vi "Trial - Rename File.vi"(11 "Current File Name":string) -> (2 "Cancel OUT":bool, 3 "Enter New File Name OUT":string caption=".dat")   [LabVIEW 2018]
panel:
  in  "Enter New File Name":string caption=".dat"
  in  "Cancel":bool
  in  "Save":bool
  # "Enter New File Name for Trial"
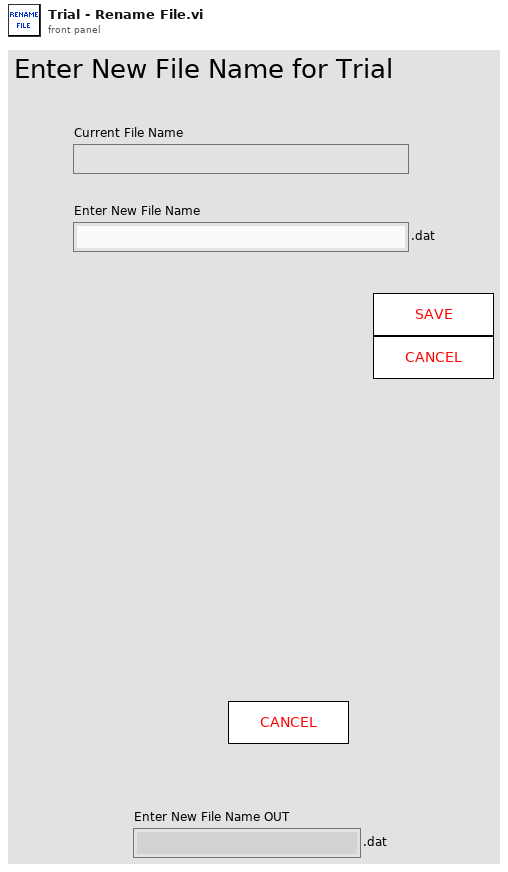
[diagram p1: front panel]
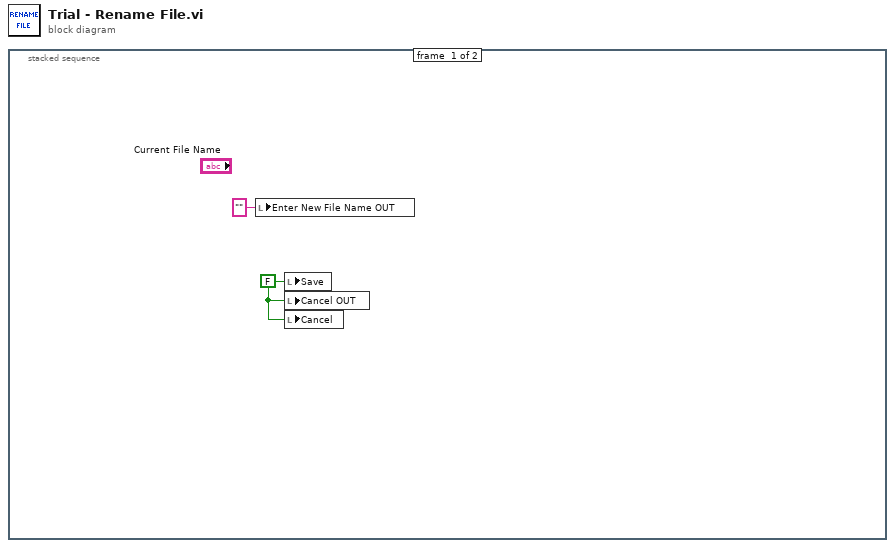
[diagram p0: block diagram]
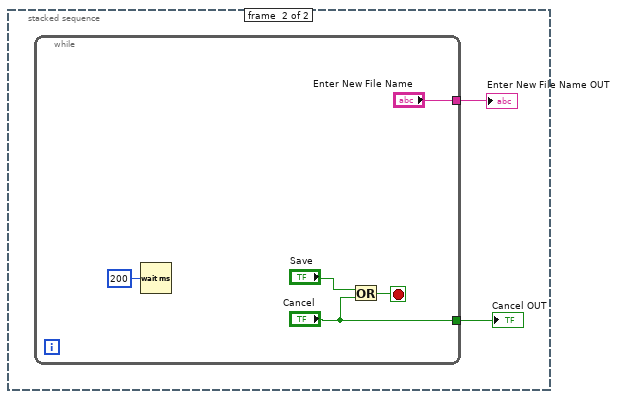
[diagram p2: hidden frame]
diagram:
  n1 = stacked-sequence {
    frame #0 {
      w2 = FALSE ("Save")
      n2 = local write "Enter New File Name OUT"("" ("Enter New File Name OUT")) -> ()
      n3 = local write "Save"(w2) -> ()
      n4 = local write "Cancel OUT"(w2) -> ()
      n5 = local write "Cancel"(w2) -> ()
    }
    frame #1 {
      n6 = while {
        tunnel: ["Cancel"] -> w4
        tunnel: ["Enter New File Name"] -> w3
        stop <- w9 stop-if-true
        n7 = Wait (ms)(milliseconds to wait=u32 200) -> ()  [unwired: 1 out]
        n8 = Or(x="Save", y="Cancel") -> (x .or. y?=w9:bool)
      }
      "Cancel OUT" <- w4
      "Enter New File Name OUT" <- w3
    }
  }
